vi "CreateNode.vi"(7 "DOM Document":refnum<k20>, 8 "Error In":errorcluster, 10 "Text":string, 11 "Tag Name":string) -> (0 "Error out":errorcluster, 3 "Node":refnum<k20>)   [LabVIEW 2013, in "LV-Utilities.lvlib"]
uses:
  LV-Utilities.lvlib
  <resource>/objmgr/DOMUserDefRef.rc
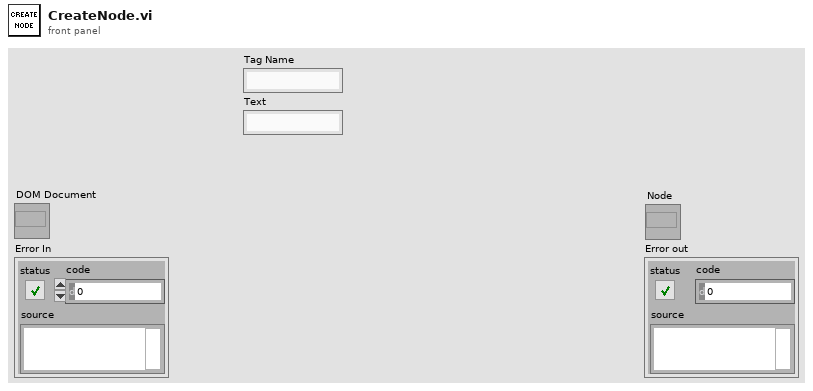
[diagram p1: front panel]
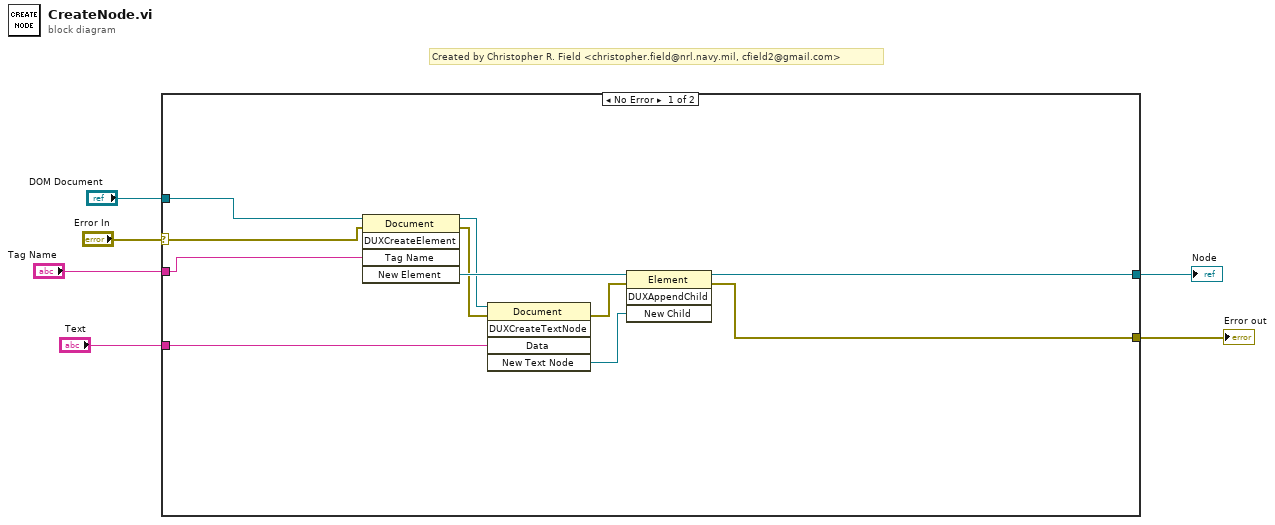
[diagram p0: block diagram]
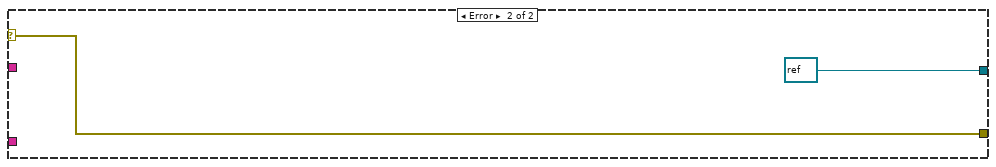
[diagram p2: hidden frame]
diagram:
  # "Created by Christopher R. Field <christopher.field@nrl.navy.mil, cfield2@gmail.com>"
  n1 = case shown="No Error" "Error In" {
    selector: "Error In" -> [w9 w19]
    tunnel: "DOM Document" -> [w17 _]
    tunnel: [w16 refnum<k20> refnum ("Operator Node 2")] -> w5
    tunnel: [w15 w19] -> w4
    tunnel: "Tag Name" -> [w8 _]
    tunnel: "Text" -> [w7 _]
    frame No Error {
      n2 = invoke class="Document" method="DUXCreateElement"(reference=w17, error in=w9, "Tag Name"=w8) -> (reference out=w13:refnum<k20>, error out=w12:errorcluster, "New Element"=w14:refnum<k20>)  [unwired: 2 in, 2 out]
      n3 = invoke class="Document" method="DUXCreateTextNode"(reference=w13, error in=w12, "Data"=w7) -> (error out=w11:errorcluster, "New Text Node"=w10:refnum<k20>)  [unwired: 2 in, 3 out]
      n4 = invoke class="Element" method="DUXAppendChild"(reference=w14, error in=w11, "New Child"=w10) -> (reference out=w16:refnum<k20>, error out=w15:errorcluster)  [unwired: 1 in, 2 out]
    }
    frame Error {
    }
  }
  "Node" <- w5
  "Error out" <- w4
